vi "Get Pressure.vi"(8 "error in (no error)":errorcluster, 9 "Pressure unit":T1(ring), 11 "Sensor General Class in":refnum<class "Sensor General Class.lvclass">) -> (0 "error out":errorcluster, 2 "Pressure":sgl, 3 "Sensor General Class out":refnum<class "Sensor General Class.lvclass">)   [LabVIEW 2020, in "Sensor General Class.lvclass"]
uses:
  Sensor General Class.lvclass
  Data Enum.ctl
  Sensor General Class.lvclass/Sensor General Class.ctl
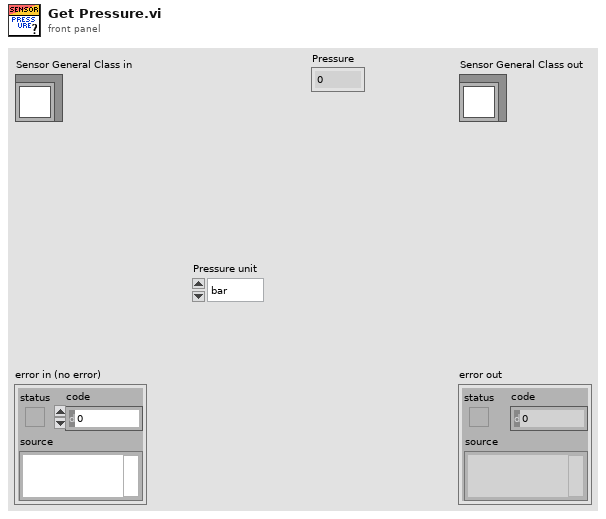
[diagram p1: front panel]
types:
  T1 = enum16{"bar", "MPa", "Pa", "kPa", "psi", "H/cm^2"}
  T2 = typedef "Sensor General Class.lvclass/Data Enum.ctl" = enum16{"p_bar", "p_MPa", "p_Pa", "p_kPa", "p_psi", "p_H/cm^2", "t_C", "t_K", "t_F", "rho_g/l", "rho_kg/m^3", "p20_bar", "related p20_bar", "p20_MPa", "related p20_MPa", "Tf_SF6", "Td_sf6", "tank Tf_SF6", "tank Td_SF6", "Tf_N2", "Td_N2", "tank Tf_N2", "tank Td_N2", "ppm_v SF6", "ppm_w SF6", "ppm_v N2", "ppm_w N2", "rH", "errors"}
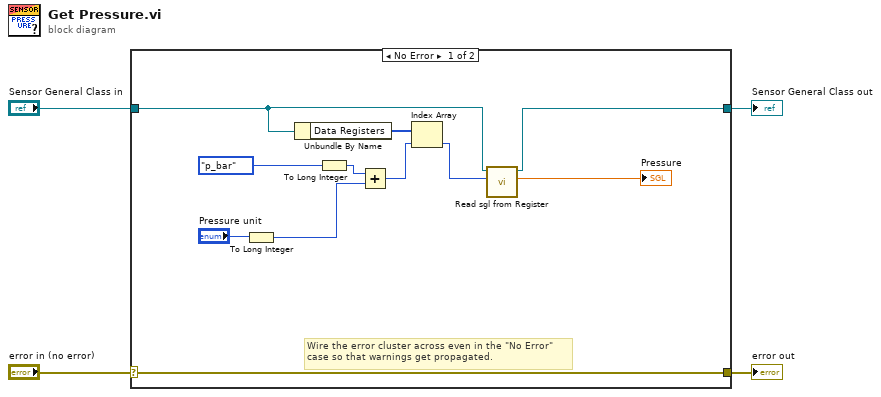
[diagram p0: block diagram]
diagram:
  n1 = case shown="No Error" "error in (no error)" {
    selector: "error in (no error)" -> [w15 w17]
    tunnel: [w15 w17] -> w3
    tunnel: [w5 w16] -> w1
    tunnel: "Sensor General Class in" -> [w6 w16]
    frame No Error {
      # "Wire the error cluster across even in the \"No Error\"\ncase so that warnings get propagated."
      n2 = To Long Integer(number="Pressure unit") -> (32bit integer=w11:i32)
      n3 = Unbundle By Name(w6) -> ("Data Registers"=w9:u16[])
      n4 = To Long Integer(number=Data_Enum."p_bar" ("Data Enum")) -> (32bit integer=w12:i32)
      n5 = Add(x=w12, y=w11) -> (x+y=w8:i32)
      n6 = Index Array(array=w9, index=w8) -> (element=w7:u16)
      n7 = call-dynamic "Read sgl from Register.vi"("Start Register"=w7, "Sensor General Class in"=w6) -> ("Data"=→"Pressure":sgl, "Sensor General Class out"=w5:refnum<class "Sensor General Class.lvclass">)  [unwired: 7 in, 1 out]
    }
    frame Error {
    }
  }
  "error out" <- w3
  "Sensor General Class out" <- w1
